vi "FlyWheelSim_Pack_Simulation_Params.vi"(11 "Vel Meas StdDev Rad/Sec":dbl=1.0) -> (3 "FlyWheelSim_Simulation_Params":T1 {"Vel Meas Std Dev Rad/Sec" format="%#_13g"})   [LabVIEW 2019, in "Trajectory_Library.lvlib"]
uses:
  Trajectory_Library.lvlib
  TypeDef/FLYWHEEL_SIM_SIMULATION_PARAMS.ctl
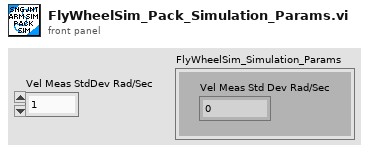
[diagram p1: front panel]
types:
  T1 = typedef "Trajectory_Library.lvlib/FLYWHEEL_SIM_SIMULATION_PARAMS.ctl" = cluster{"Vel Meas Std Dev Rad/Sec":dbl}
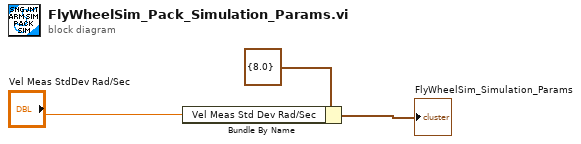
[diagram p0: block diagram]
diagram:
  n1 = Bundle By Name(cluster=T1 {"Vel Meas Std Dev Rad/Sec"=8.0} ("FlyWheelSim_Simulation_Params"), "Vel Meas Std Dev Rad/Sec"="Vel Meas StdDev Rad/Sec") -> (→"FlyWheelSim_Simulation_Params":T1)
